vi "Send Command Query (non-enum).vi"(8 "error in (no error)":errorcluster, 10 "Command":string, 11 "Laser in":refnum<class "Laser.lvclass">) -> (0 "error out":errorcluster, 2 "Response":string, 3 "Laser out":refnum<class "Laser.lvclass">)   [LabVIEW 2018, in "Laser.lvlib" / "Laser.lvclass"]
doc: "This Override is used to send a command to the targeted device and read the reponse\nNOTE: This Override was created to provide means to sends commands that are not part of the Command LIst.ctl whic was initially intended for Model H Laser (Kronos)"
uses:
  Laser.lvclass
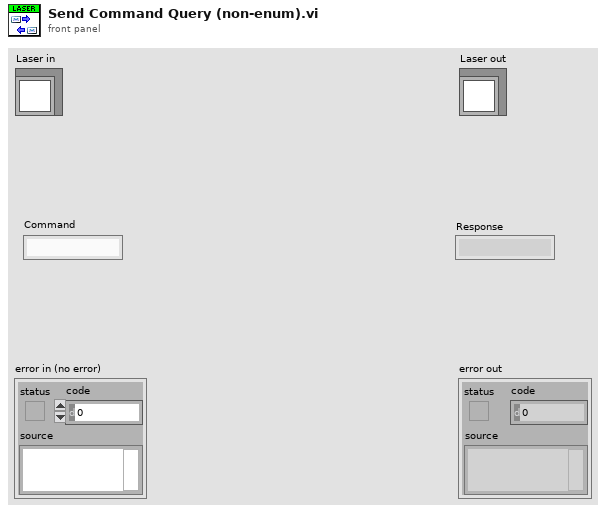
[diagram p1: front panel]
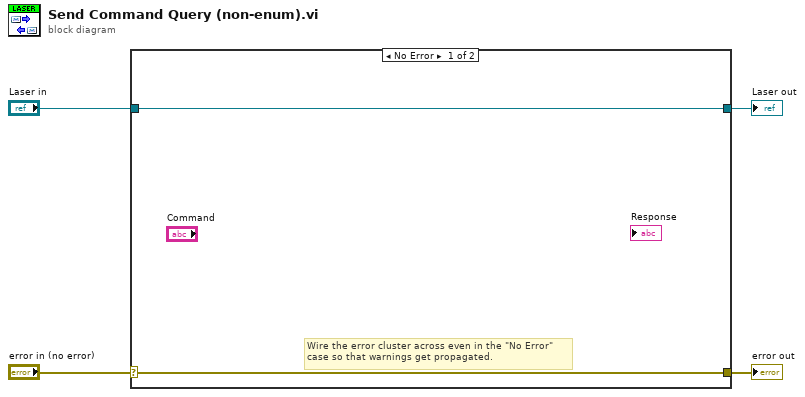
[diagram p0: block diagram]
diagram:
  n1 = case shown="No Error" "error in (no error)" {
    selector: "error in (no error)" -> [w5 w8]
    tunnel: [w5 w8] -> w3
    tunnel: [w6 w7] -> w1
    tunnel: "Laser in" -> [w6 w7]
    frame No Error {
      # "Wire the error cluster across even in the \"No Error\"\ncase so that warnings get propagated."
    }
    frame Error {
    }
  }
  "error out" <- w3
  "Laser out" <- w1
